vi "inflation_deflation.vi"() -> ()   [LabVIEW 2014]
uses:
  <vilib>/vision/NI_Vision_Development_Module.lvlib
  <instrlib>/KD Scientific 2XX Series/KD Scientific 2XX Series.lvlib
panel:
  in  "Default Pressure":dbl
  out "Absolute Difference":dbl
  in  "stop 3":bool
  in  "Number of Cycles":i32
  in  "Min Pressure":dbl
  in  "Max Pressure":dbl
  out "Status":T1
  in  "stop 2":bool
  out "Delivered Volume":dbl
  out "Units":string
  in  "Baud Rate (9600)":u32(ring)=9600 items=["300"=300, "1200"=1200, "2400"=2400, "4800"=4800, "9600"=9600]
  in  "Withdrawal Settings":T2={"Flow Rate (5)"=5.0, "Volume (10)"=10.0, "Volume Units (ml)"=enum."milliliters (ml)", "Rate Units (ml/min.)"=enum."milliliters per minute (ml/min.)"} {"Volume (10)" format="%#.3g"}
  in  "Diameter (29.5 mm)":dbl=8.75
  in  "Infusion Settings":T2={"Flow Rate (5)"=5.0, "Volume (10)"=10.0, "Volume Units (ml)"=enum."milliliters (ml)", "Rate Units (ml/min.)"=enum."milliliters per minute (ml/min.)"}
  in  "Address (0)":i32 format="%0.0f"
  in  "error in (no error)":errorcluster
  in  "VISA resource name (4)":refnum<visa-resource-name>="COM1"
  in  "stop":bool
  out "Image":T3(plugin-control)
  out "Particle Measurements (Pixels) (Particle Analysis 1)":dbl[][](array[numeric]) format="%.2f"
  out "subarray":dbl[](array[numeric])
  out "The diameter":dbl[](array[numeric])
  in  "stop (F)":bool
  out "Data from Transducer":dynamicdata(graph) caption="Voltage from Transducer V"
  out "Voltage from pressure transducer":dbl[](array[numeric])
  out "Pressure mm Hg":dbl[](graph)
  in  "Calibration factor(-25.53)":dbl[](array[numeric])
  in  "Zero Error(-.09)":dbl[](array[numeric])
  out "pressure mm Hg":dbl[](array[numeric])
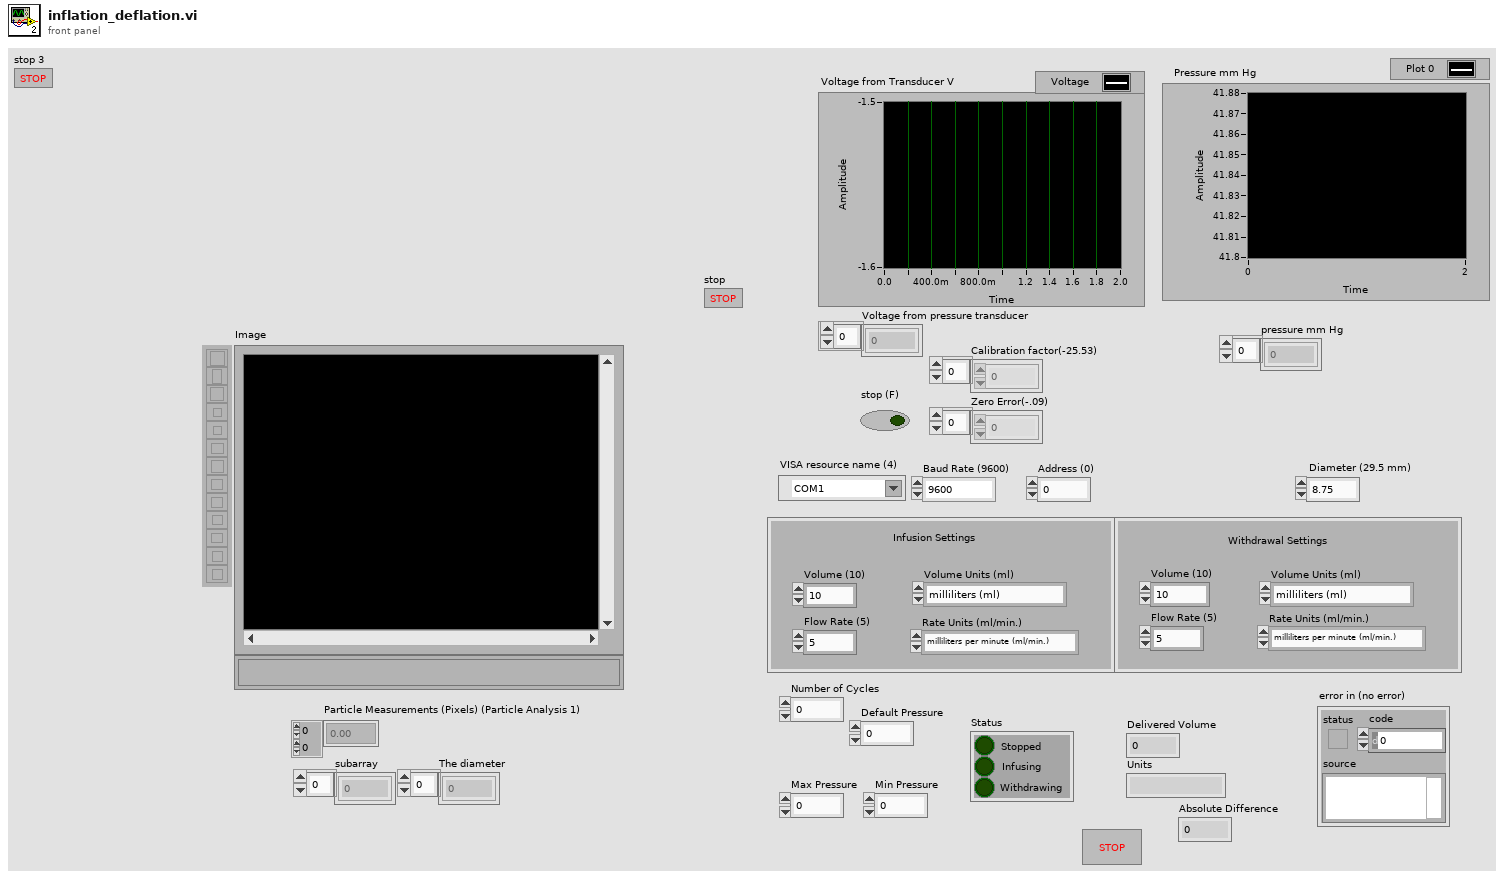
[diagram p1: front panel]
types:
  T1 = cluster{"Stopped":bool, "Infusing":bool, "Withdrawing":bool}
  T2 = cluster{"Flow Rate (5)":dbl, "Volume (10)":dbl, "Volume Units (ml)":enum16{"milliliters (ml)", "microliters (ul)"}, "Rate Units (ml/min.)":enum16{"milliliters per minute (ml/min.)", "milliliters per hour (ml/hr.)", "microliters per minute (ul/min.)", "microliters per hour (ul/hr.)"}}
  T3 = typedef "IMAQ Image.ctl" = refnum<image>
  T4 = typedef "Board Id" = u8
  T5 = typedef "ROI Descriptor" = cluster{"Global Rectangle":i32[], "Contours":cluster{"ID":enum32{"External", "Internal"}, "Type":u32, "Coordinates":i32[]}[]}
  T6 = enum16{"milliliters per minute (ml/min.)", "milliliters per hour (ml/hr.)", "microliters per minute (ul/min.)", "microliters per hour (ul/hr.)"}
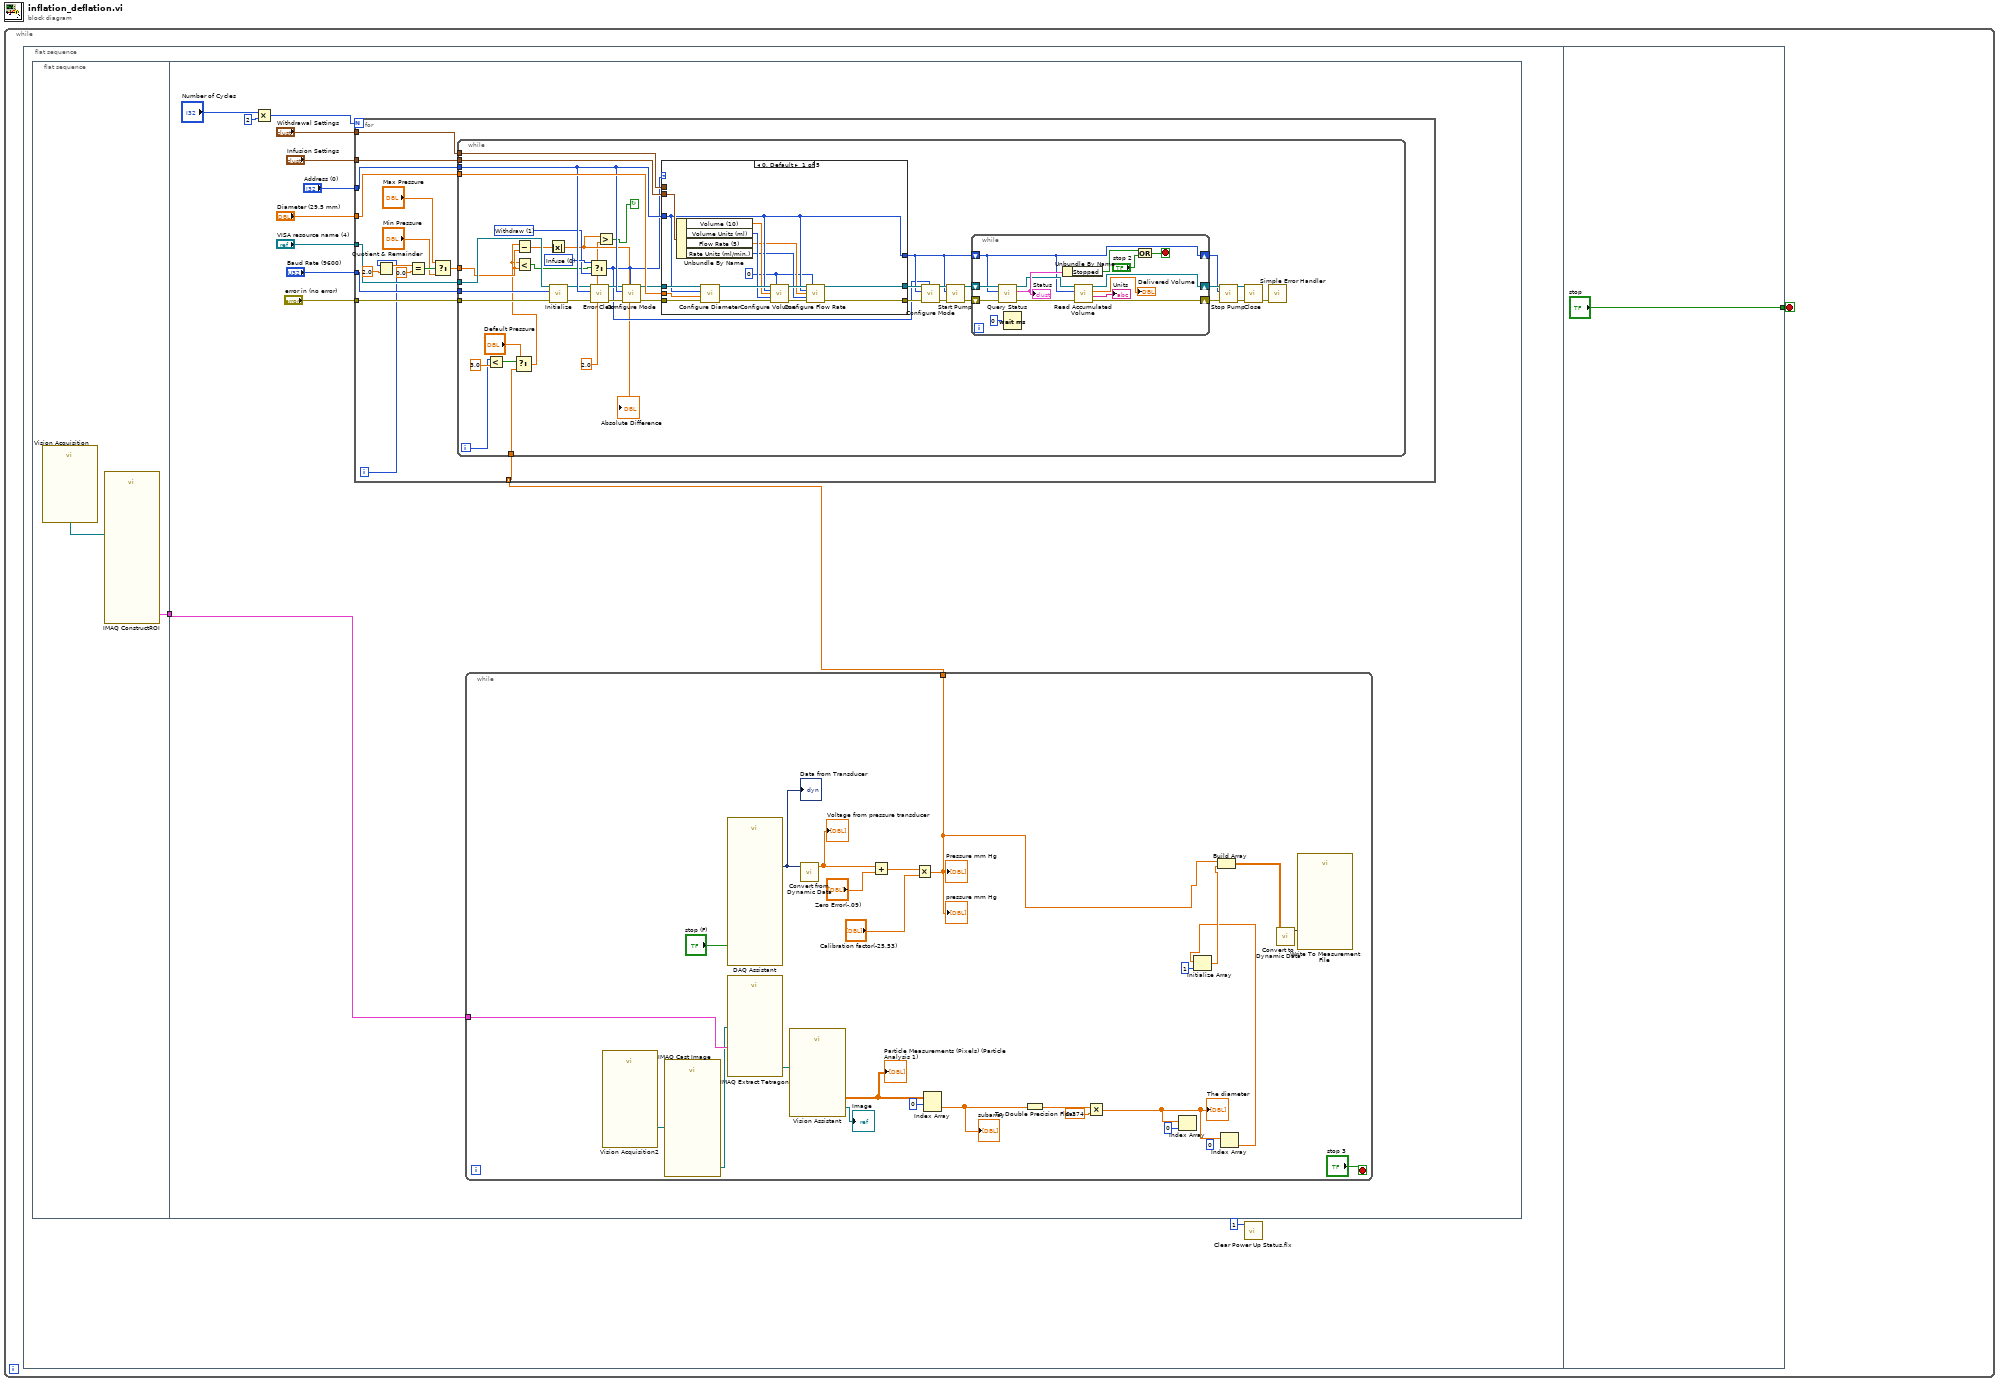
[diagram p0: block diagram]
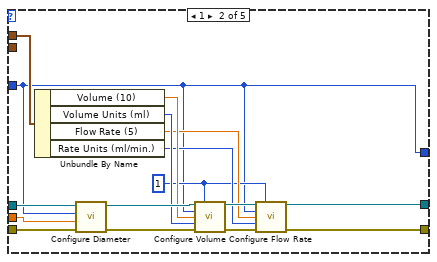
[diagram p2: hidden frame]
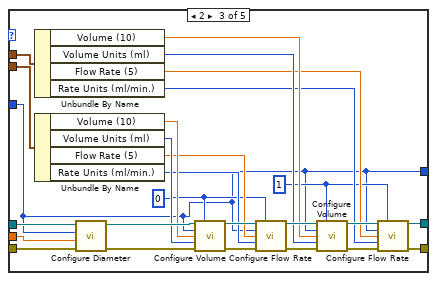
[diagram p3: hidden frame]
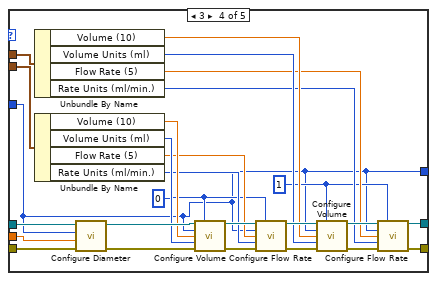
[diagram p4: hidden frame]
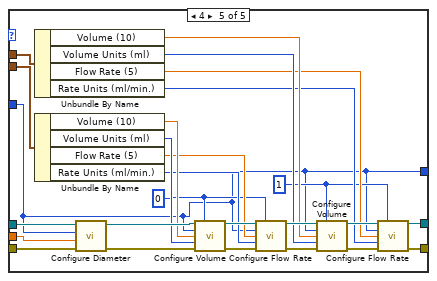
[diagram p5: hidden frame]
diagram:
  n1 = while {
    stop <- w1 stop-if-true
    n2 = flat-sequence {
      tunnel: ["stop"] -> w1
      frame #0 {
        n3 = flat-sequence {
          tunnel: [w4] -> w3
          tunnel: w3 -> [w8]
          frame #0 {
            n4 = call "Vision Acquisition"() -> ("Image Out"=w5:T3)  [unwired: 26 in, 1 out]
            n5 = call "IMAQ ConstructROI"("Image"=w5) -> ("ROI Descriptor Out"=w4:T5)  [unwired: 7 in, 3 out]
          }
          frame #1 {
            n6 = Multiply(x="Number of Cycles", y=2) -> (x*y=w7:i32)
            n7 = while {
              tunnel: w8 -> [w42]
              tunnel: [w20] -> w6
              stop <- "stop 3" stop-if-true
              (unwired) 0 ("index")
              n8 = call "Vision Acquisition2"() -> ("Image Out"=w29:T3)  [unwired: 25 in, 2 out]
              n9 = call "IMAQ Cast Image"("Image Src"=w29) -> ("Image Dst Out"=w19:T3)  [unwired: 9 in, 1 out]
              n10 = call "DAQ Assistant"("stop (F)"="stop (F)") -> ("data"=w27:dynamicdata)  [unwired: 15 in, 3 out]
              "Data from Transducer" <- w27
              n11 = call-poly "IMAQ Extract Tetragon"("ROI Descriptor"=w42, "Image Src"=w19) -> ("Image Dst Out"=w36:T3)  [unwired: 8 in, 1 out]
              n12 = call "Vision Assistant"("Image In"=w36) -> ("Image Out"=→"Image":T3, "Particle Measurements (Pixels) (Particle Analysis 1)"=w35:dbl[][])  [unwired: 23 in, 2 out]
              "Particle Measurements (Pixels) (Particle Analysis 1)" <- w35
              n13 = call "Convert from Dynamic Data"("Dynamic Data Type"=w27) -> ("Array"=w24:dbl[])  [unwired: 3 in]
              "Voltage from pressure transducer" <- w24
              n14 = Add(x=w24, y="Zero Error(-.09)") -> (x+y=w26:dbl[])
              n15 = Multiply(x=w26, y="Calibration factor(-25.53)") -> (x*y=w20:dbl[])
              "Pressure mm Hg" <- w20
              "pressure mm Hg" <- w20
              n16 = Index Array(array=w35, index (row)=0) -> (element=w33:dbl[])  [unwired: 1 in]
              "subarray" <- w33
              n17 = To Double Precision Float(number=w33) -> (double precision float=w32:dbl[])
              n18 = Multiply(x=w32, y=0.374) -> (x*y=w28:dbl[])
              "The diameter" <- w28
              n19 = Index Array(array=w28, index=0) -> ()  [unwired: 1 out]
              n20 = Index Array(array=w28) -> (element=w21:dbl)  [unwired: 1 in]
              n21 = Initialize Array(w21, 1 ("dimension size")) -> (w39:dbl[])
              n22 = Build Array(w20, w39) -> (w40:dbl[][])
              n23 = call "Convert to Dynamic Data"("2D Array"=w40) -> ("Dynamic Data Type"=w41:dynamicdata)  [unwired: 3 in]
              n24 = call "Write To Measurement File"("Signals"=w41) -> ()  [unwired: 16 in, 3 out]
            }
            n25 = for {
              N: w7 -> [_]
              tunnel: "Address (0)" -> [w58]
              tunnel: "Baud Rate (9600)" -> [w57]
              tunnel: "Diameter (29.5 mm)" -> [w56]
              tunnel: "Withdrawal Settings" -> [w55]
              tunnel: "Infusion Settings" -> [w54]
              tunnel: "error in (no error)" -> [w53]
              tunnel: "VISA resource name (4)" -> [w52]
              tunnel: w6 -> [w44] mode=indexing
              i -> [w43]
              n26 = Quotient & Remainder(x=w43, y=2.0) -> (x-y*floor(x/y)=w49:dbl)  [unwired: 1 out]
              n27 = Equal?(x=w49, y=0.0) -> (x = y?=w48:bool)
              n28 = Select(t="Max Pressure", s=w48, f="Min Pressure") -> (s? t:f=w45:dbl)
              n29 = while {
                tunnel: w52 -> [w99]
                tunnel: w53 -> [w98]
                tunnel: w54 -> [w97]
                tunnel: w55 -> [w96]
                tunnel: w56 -> [w95]
                tunnel: w57 -> [w94]
                tunnel: w58 -> [w93]
                tunnel: w45 -> [w70]
                tunnel: w44 -> [w60]
                i -> [w63]
                stop <- w65 continue-if-true
                w72 = u16 1 items=["Withdraw"=1]
                w73 = u16 0 items=["Infuse"] ("Mode (infuse)")
                n30 = Less?(x=w63, y=3.0) -> (x < y?=w62:bool)
                n31 = Select(t="Default Pressure", s=w62, f=w60) -> (s? t:f=w59:dbl)
                n32 = Subtract(x=w59, y=w70) -> (x-y=w69:dbl)
                n33 = Less?(x=w59, y=w70) -> (x < y?=w66:bool)
                n34 = Absolute Value(x=w69) -> (abs(x)=w68:dbl)
                "Absolute Difference" <- w68
                n35 = call <instrlib>:"Initialize.vi"("error in (no error)"=w98, "Baud Rate (9600)"=w94, "VISA resource name"=w99) -> ("error out"=w75:errorcluster, "VISA resource name out"=w74:refnum<visa-resource-name>)  [unwired: 7 in]
                n36 = Select(t=w73, s=w66, f=w72) -> (s? t:f=w71:u16)
                n37 = call <instrlib>:"Error Clear.vi"("error in (no error)"=w75, "Address (0)"=w93, "VISA resource name"=w74) -> ("error out"=w76:errorcluster, "VISA resource name out"=w77:refnum<visa-resource-name>)  [unwired: 6 in, 1 out]
                n38 = Greater?(x=w68, y=2.0) -> (0:w65:bool)
                n39 = call <instrlib>:"Configure Mode.vi"("Mode (infuse)"=w71, "error in (no error)"=w76, "Address (0)"=w93, "VISA resource name"=w77) -> ("error out"=w79:errorcluster, "VISA resource name out"=w78:refnum<visa-resource-name>)  [unwired: 6 in]
                n40 = case shown="0, Default" w71 {
                  tunnel: w97 -> [w109 _ w157 w183 w209]
                  tunnel: w96 -> [_ w131 w156 w182 w208]
                  tunnel: w78 -> [w115 w130 w155 w181 w207]
                  tunnel: w79 -> [w114 w126 w154 w180 w206]
                  tunnel: w95 -> [w108 w122 w137 w163 w189]
                  tunnel: [w107 w116 w132 w158 w184] -> w80
                  tunnel: w93 -> [w107 w116 w132 w158 w184]
                  tunnel: [w102 w127 w134 w160 w186] -> w84
                  tunnel: [w101 w123 w133 w159 w185] -> w83
                  frame 0, Default {
                    w100 = 0
                    n41 = Unbundle By Name(w109) -> ("Volume (10)"=w106:dbl, "Volume Units (ml)"=w105:enum16{"milliliters (ml)", "microliters (ul)"}, "Flow Rate (5)"=w104:dbl, "Rate Units (ml/min.)"=w103:T6)
                    n42 = call <instrlib>:"Configure Diameter.vi"("error in (no error)"=w114, "Diameter (8.75 mm)"=w108, "Address (0)"=w107, "VISA resource name"=w115) -> ("error out"=w112:errorcluster, "VISA resource name out"=w113:refnum<visa-resource-name>)  [unwired: 6 in]
                    n43 = call <instrlib>:"Configure Volume.vi"("VISA resource name"=w113, "Mode (infuse)"=w100, "Address (0)"=w107, "Volume (100)"=w106, "Units (0: milliliters)"=w105, "error in (no error)"=w112) -> ("VISA resource name out"=w111:refnum<visa-resource-name>, "error out"=w110:errorcluster)  [unwired: 8 in]
                    n44 = call <instrlib>:"Configure Flow Rate.vi"("VISA resource name"=w111, "Mode (infuse)"=w100, "Address (0)"=w107, "Flow Rate (5)"=w104, "Units (0: milliliters per minute)"=w103, "error in (no error)"=w110) -> ("VISA resource name out"=w102:refnum<visa-resource-name>, "error out"=w101:errorcluster)  [unwired: 8 in]
                  }
                  frame 1 {
                    w117 = 1
                    n45 = Unbundle By Name(w131) -> ("Volume (10)"=w121:dbl, "Volume Units (ml)"=w120:enum16{"milliliters (ml)", "microliters (ul)"}, "Flow Rate (5)"=w119:dbl, "Rate Units (ml/min.)"=w118:T6)
                    n46 = call <instrlib>:"Configure Diameter.vi"("error in (no error)"=w126, "Diameter (8.75 mm)"=w122, "Address (0)"=w116, "VISA resource name"=w130) -> ("error out"=w125:errorcluster, "VISA resource name out"=w129:refnum<visa-resource-name>)  [unwired: 6 in]
                    n47 = call <instrlib>:"Configure Volume.vi"("VISA resource name"=w129, "Mode (infuse)"=w117, "Address (0)"=w116, "Volume (100)"=w121, "Units (0: milliliters)"=w120, "error in (no error)"=w125) -> ("VISA resource name out"=w128:refnum<visa-resource-name>, "error out"=w124:errorcluster)  [unwired: 8 in]
                    n48 = call <instrlib>:"Configure Flow Rate.vi"("VISA resource name"=w128, "Mode (infuse)"=w117, "Address (0)"=w116, "Flow Rate (5)"=w119, "Units (0: milliliters per minute)"=w118, "error in (no error)"=w124) -> ("VISA resource name out"=w127:refnum<visa-resource-name>, "error out"=w123:errorcluster)  [unwired: 8 in]
                  }
                  frame 2 {
                    w135 = 1
                    w136 = 0
                    n49 = Unbundle By Name(w156) -> ("Volume (10)"=w141:dbl, "Volume Units (ml)"=w140:enum16{"milliliters (ml)", "microliters (ul)"}, "Flow Rate (5)"=w139:dbl, "Rate Units (ml/min.)"=w138:T6)
                    n50 = Unbundle By Name(w157) -> ("Volume (10)"=w145:dbl, "Volume Units (ml)"=w144:enum16{"milliliters (ml)", "microliters (ul)"}, "Flow Rate (5)"=w143:dbl, "Rate Units (ml/min.)"=w142:T6)
                    n51 = call <instrlib>:"Configure Diameter.vi"("error in (no error)"=w154, "Diameter (8.75 mm)"=w137, "Address (0)"=w132, "VISA resource name"=w155) -> ("error out"=w149:errorcluster, "VISA resource name out"=w153:refnum<visa-resource-name>)  [unwired: 6 in]
                    n52 = call <instrlib>:"Configure Volume.vi"("VISA resource name"=w153, "Mode (infuse)"=w136, "Address (0)"=w132, "Volume (100)"=w145, "Units (0: milliliters)"=w144, "error in (no error)"=w149) -> ("VISA resource name out"=w152:refnum<visa-resource-name>, "error out"=w148:errorcluster)  [unwired: 8 in]
                    n53 = call <instrlib>:"Configure Flow Rate.vi"("VISA resource name"=w152, "Mode (infuse)"=w136, "Address (0)"=w132, "Flow Rate (5)"=w143, "Units (0: milliliters per minute)"=w142, "error in (no error)"=w148) -> ("VISA resource name out"=w151:refnum<visa-resource-name>, "error out"=w147:errorcluster)  [unwired: 8 in]
                    n54 = call <instrlib>:"Configure Volume.vi"("VISA resource name"=w151, "Mode (infuse)"=w135, "Address (0)"=w132, "Volume (100)"=w141, "Units (0: milliliters)"=w140, "error in (no error)"=w147) -> ("VISA resource name out"=w150:refnum<visa-resource-name>, "error out"=w146:errorcluster)  [unwired: 8 in]
                    n55 = call <instrlib>:"Configure Flow Rate.vi"("VISA resource name"=w150, "Mode (infuse)"=w135, "Address (0)"=w132, "Flow Rate (5)"=w139, "Units (0: milliliters per minute)"=w138, "error in (no error)"=w146) -> ("VISA resource name out"=w134:refnum<visa-resource-name>, "error out"=w133:errorcluster)  [unwired: 8 in]
                  }
                  frame 3 {
                    w161 = 1
                    w162 = 0
                    n56 = Unbundle By Name(w182) -> ("Volume (10)"=w167:dbl, "Volume Units (ml)"=w166:enum16{"milliliters (ml)", "microliters (ul)"}, "Flow Rate (5)"=w165:dbl, "Rate Units (ml/min.)"=w164:T6)
                    n57 = Unbundle By Name(w183) -> ("Volume (10)"=w171:dbl, "Volume Units (ml)"=w170:enum16{"milliliters (ml)", "microliters (ul)"}, "Flow Rate (5)"=w169:dbl, "Rate Units (ml/min.)"=w168:T6)
                    n58 = call <instrlib>:"Configure Diameter.vi"("error in (no error)"=w180, "Diameter (8.75 mm)"=w163, "Address (0)"=w158, "VISA resource name"=w181) -> ("error out"=w175:errorcluster, "VISA resource name out"=w179:refnum<visa-resource-name>)  [unwired: 6 in]
                    n59 = call <instrlib>:"Configure Volume.vi"("VISA resource name"=w179, "Mode (infuse)"=w162, "Address (0)"=w158, "Volume (100)"=w171, "Units (0: milliliters)"=w170, "error in (no error)"=w175) -> ("VISA resource name out"=w178:refnum<visa-resource-name>, "error out"=w174:errorcluster)  [unwired: 8 in]
                    n60 = call <instrlib>:"Configure Flow Rate.vi"("VISA resource name"=w178, "Mode (infuse)"=w162, "Address (0)"=w158, "Flow Rate (5)"=w169, "Units (0: milliliters per minute)"=w168, "error in (no error)"=w174) -> ("VISA resource name out"=w177:refnum<visa-resource-name>, "error out"=w173:errorcluster)  [unwired: 8 in]
                    n61 = call <instrlib>:"Configure Volume.vi"("VISA resource name"=w177, "Mode (infuse)"=w161, "Address (0)"=w158, "Volume (100)"=w167, "Units (0: milliliters)"=w166, "error in (no error)"=w173) -> ("VISA resource name out"=w176:refnum<visa-resource-name>, "error out"=w172:errorcluster)  [unwired: 8 in]
                    n62 = call <instrlib>:"Configure Flow Rate.vi"("VISA resource name"=w176, "Mode (infuse)"=w161, "Address (0)"=w158, "Flow Rate (5)"=w165, "Units (0: milliliters per minute)"=w164, "error in (no error)"=w172) -> ("VISA resource name out"=w160:refnum<visa-resource-name>, "error out"=w159:errorcluster)  [unwired: 8 in]
                  }
                  frame 4 {
                    w187 = 1
                    w188 = 0
                    n63 = Unbundle By Name(w208) -> ("Volume (10)"=w193:dbl, "Volume Units (ml)"=w192:enum16{"milliliters (ml)", "microliters (ul)"}, "Flow Rate (5)"=w191:dbl, "Rate Units (ml/min.)"=w190:T6)
                    n64 = Unbundle By Name(w209) -> ("Volume (10)"=w197:dbl, "Volume Units (ml)"=w196:enum16{"milliliters (ml)", "microliters (ul)"}, "Flow Rate (5)"=w195:dbl, "Rate Units (ml/min.)"=w194:T6)
                    n65 = call <instrlib>:"Configure Diameter.vi"("error in (no error)"=w206, "Diameter (8.75 mm)"=w189, "Address (0)"=w184, "VISA resource name"=w207) -> ("error out"=w201:errorcluster, "VISA resource name out"=w205:refnum<visa-resource-name>)  [unwired: 6 in]
                    n66 = call <instrlib>:"Configure Volume.vi"("VISA resource name"=w205, "Mode (infuse)"=w188, "Address (0)"=w184, "Volume (100)"=w197, "Units (0: milliliters)"=w196, "error in (no error)"=w201) -> ("VISA resource name out"=w204:refnum<visa-resource-name>, "error out"=w200:errorcluster)  [unwired: 8 in]
                    n67 = call <instrlib>:"Configure Flow Rate.vi"("VISA resource name"=w204, "Mode (infuse)"=w188, "Address (0)"=w184, "Flow Rate (5)"=w195, "Units (0: milliliters per minute)"=w194, "error in (no error)"=w200) -> ("VISA resource name out"=w203:refnum<visa-resource-name>, "error out"=w199:errorcluster)  [unwired: 8 in]
                    n68 = call <instrlib>:"Configure Volume.vi"("VISA resource name"=w203, "Mode (infuse)"=w187, "Address (0)"=w184, "Volume (100)"=w193, "Units (0: milliliters)"=w192, "error in (no error)"=w199) -> ("VISA resource name out"=w202:refnum<visa-resource-name>, "error out"=w198:errorcluster)  [unwired: 8 in]
                    n69 = call <instrlib>:"Configure Flow Rate.vi"("VISA resource name"=w202, "Mode (infuse)"=w187, "Address (0)"=w184, "Flow Rate (5)"=w191, "Units (0: milliliters per minute)"=w190, "error in (no error)"=w198) -> ("VISA resource name out"=w186:refnum<visa-resource-name>, "error out"=w185:errorcluster)  [unwired: 8 in]
                  }
                }
                n70 = call <instrlib>:"Configure Mode.vi"("Mode (infuse)"=w71, "error in (no error)"=w83, "Address (0)"=w80, "VISA resource name"=w84) -> ("error out"=w81:errorcluster, "VISA resource name out"=w82:refnum<visa-resource-name>)  [unwired: 6 in]
                n71 = call <instrlib>:"Start Pump.vi"("error in (no error)"=w81, "Address (0)"=w80, "VISA resource name"=w82) -> ("error out"=w91:errorcluster, "VISA resource name out"=w92:refnum<visa-resource-name>)  [unwired: 7 in]
                n72 = while {
                  shift-right: [w212] -> w88
                  shift-left: w80 -> [w212]
                  shift-right: [w214] -> w90
                  shift-left: w92 -> [w220]
                  shift-right: [w213] -> w89
                  shift-left: w91 -> [w221]
                  stop <- w218 stop-if-true
                  n73 = call <instrlib>:"Query Status.vi"("error in (no error)"=w221, "Address (0)"=w212, "VISA resource name"=w220) -> ("error out"=w223:errorcluster, "Status"=w219:T1, "VISA resource name out"=w215:refnum<visa-resource-name>)  [unwired: 6 in]
                  "Status" <- w219
                  n74 = Wait (ms)(milliseconds to wait=u32 0) -> ()  [unwired: 1 out]
                  n75 = Unbundle By Name(w219) -> ("Stopped"=w217:bool)
                  n76 = call <instrlib>:"Read Accumulated Volume.vi"("error in (no error)"=w223, "Address (0)"=w212, "VISA resource name"=w215) -> ("error out"=w213:errorcluster, "Units"=→"Units":string, "Delivered Volume"=→"Delivered Volume":dbl, "VISA resource name out"=w214:refnum<visa-resource-name>)  [unwired: 5 in]
                  n77 = Or(x=w217, y="stop 2") -> (x .or. y?=w218:bool)
                }
                n78 = call <instrlib>:"Stop Pump.vi"("error in (no error)"=w89, "Address (0)"=w88, "VISA resource name"=w90) -> ("error out"=w86:errorcluster, "VISA resource name out"=w85:refnum<visa-resource-name>)  [unwired: 7 in]
                n79 = call <instrlib>:"Close.vi"("error in (no error)"=w86, "VISA resource name"=w85) -> ("error out"=w87:errorcluster)  [unwired: 9 in]
                n80 = call <vilib>:"Simple Error Handler.vi"("error in (no error)"=w87) -> ()  [unwired: 4 in, 5 out]
              }
            }
          }
        }
        n81 = call <vilib>:"Clear Power Up Status.flx"("Board ID"=T4 1) -> ()  [unwired: 6 in, 2 out]
      }
      frame #1 {
      }
    }
  }
